vi "Launcher.vi"   [LabVIEW 2020]
uses:
  <vilib>/Astemes/Triarc Framework/Process/Process.lvclass
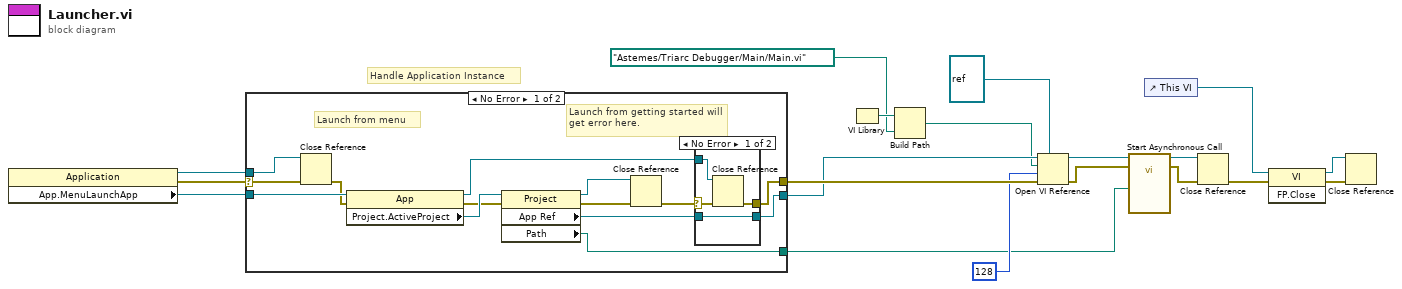
[diagram p0: block diagram]
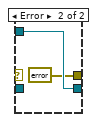
[diagram p2: hidden frame]
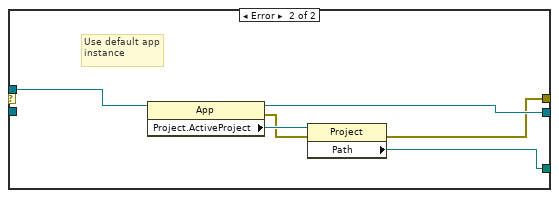
[diagram p3: hidden frame]
diagram:
  # "Handle Application Instance"
  n1 = property class="Application"() -> (reference out=w17:refnum<vi>, error out=w18:errorcluster, "App.MenuLaunchApp"=w19:refnum<vi>)  [unwired: 2 in]
  n2 = case shown="No Error" w18 {
    selector: w18 -> [w32 _]
    tunnel: [w25 w42] -> w7
    tunnel: w19 -> [w30 _]
    tunnel: w17 -> [w33 w43]
    tunnel: [w21 w41] -> w16
    tunnel: [w20 w40] -> w6
    frame No Error {
      # "Launch from getting started will get error here."
      # "Launch from menu"
      n3 = Close Reference(reference=w33, error in (no error)=w32) -> (error out=w29:errorcluster)
      n4 = property class="App"(reference=w30, error in=w29) -> (reference out=w28:refnum<vi>, error out=w26:errorcluster, "Project.ActiveProject"=w31:refnum<vi>)
      n5 = property class="Project"(reference=w31, error in=w26) -> (reference out=w27:refnum<vi>, error out=w23:errorcluster, "App Ref"=w24:refnum<vi>, "Path"=w20:path)
      n6 = Close Reference(reference=w27, error in (no error)=w23) -> (error out=w22:errorcluster)
      n7 = case shown="No Error" w22 {
        selector: w22 -> [w36 _]
        tunnel: w28 -> [w37 w39]
        tunnel: [w35 errorcluster {"status"=FALSE, "code"=0, "source"=""} ("error out")] -> w21
        tunnel: [w34 w39] -> w25
        tunnel: w24 -> [w34 _]
        frame No Error {
          n8 = Close Reference(reference=w37, error in (no error)=w36) -> (error out=w35:errorcluster)
        }
        frame Error {
        }
      }
    }
    frame Error {
      # "Use default app instance"
      n9 = property class="App"(reference=w43) -> (reference out=w42:refnum<vi>, error out=w44:errorcluster, "Project.ActiveProject"=w45:refnum<vi>)  [unwired: 1 in]
      n10 = property class="Project"(reference=w45, error in=w44) -> (error out=w41:errorcluster, "Path"=w40:path)  [unwired: 1 out]
    }
  }
  n11 = VI Library() -> (path=w5:path)
  n12 = Build Path(base path=w5, name or relative path=path "Astemes/Triarc Debugger/Main/Main.vi") -> (appended path=w3:path)
  n13 = Open VI Reference(type specifier VI Refnum (for type only)=refnum<vi> refnum, application reference (local)=w7, vi path=w3, options=128, error in (no error)=w16) -> (vi reference=w1:refnum<vi>, error out=w14:errorcluster)  [unwired: 1 in]
  n14 = call-by-ref "Start Asynchronous Call"(reference=w1, error in=w14, "Active Project"=w6) -> (reference out=w12:refnum<vi>, error out=w13:errorcluster)  [unwired: 11 in]
  n15 = control-ref of="This VI"() -> (w10:refnum<vi>)
  n16 = Close Reference(reference=w12, error in (no error)=w13) -> (error out=w11:errorcluster)
  n17 = invoke class="VI" method="FP.Close"(reference=w10, error in=w11) -> (reference out=w8:refnum<vi>, error out=w9:errorcluster)  [unwired: 1 in, 1 out]
  n18 = Close Reference(reference=w8, error in (no error)=w9) -> ()  [unwired: 1 out]
